vi "Perform Action.vi"(8 "error in":errorcluster, 10 "Input":variant, 11 "AI DAQmx Cont CFG in":refnum<class "AI Current DAQmx Cont CFG.lvclass">) -> (0 "error out":errorcluster, 2 "Output":variant, 3 "AI DAQmx Cont CFG out":refnum<class "AI Current DAQmx Cont CFG.lvclass">)   [LabVIEW 2023, in "AI Current DAQmx Cont CFG.lvclass"]
uses:
  AI Current DAQmx Cont CFG.lvclass
  D:/git/HAL/HAL GOOP4/Configuration/Configuration Semaphore/CFG Semaphore.lvclass
  D:/git/HAL/HAL GOOP4/DAQmx/DAQmx BufferLastReadsDBL/DAQmx BufferLastReadsDBL.lvclass
  D:/git/HAL/HAL GOOP4/DAQmx/DAQmx Base CFG/DAQmx Base CFG.lvclass
  Configuration/Configuration Semaphore/CFG Semaphore.lvclass/CFG Semaphore.ctl
  DAQmx/DAQmx BufferLastReadsDBL/DAQmx BufferLastReadsDBL.lvclass/DAQmx BufferLastReadsDBL.ctl
  DAQmx/DAQmx Base CFG/DAQmx Base CFG.lvclass/DAQmx Base CFG.ctl
  b39270a5-b1fd-40eb-856a-27ea7d92f2a4.vi
  <vilib>/DAQmx/read.llb/DAQmx Read (Analog 2D DBL NChan NSamp).vi
  <vilib>/JDP Science/JSONtext/Find Item.vi
  <vilib>/JDP Science/JSONtext/Next JSON Value.vi
  <vilib>/JDP Science/JSONtext/String Subset.vi
  <vilib>/JDP Science/JSONtext/Parsing/Advance past next JSON Value (inlined COPY).vi
  <vilib>/JDP Science/JSONtext/Parsing/Advance past whitespace.vi
  <vilib>/JDP Science/JSONtext/Parsing/Advance past String.vi
  <vilib>/JDP Science/JSONtext/Parsing/Advance past Number.vi
  <vilib>/JDP Science/JSONtext/Parsing/Advance past Line Ending.vi
  <vilib>/JDP Science/JSONtext/Parsing/Parse Full Path or Item Name.vi
  <vilib>/JDP Science/JSONtext/Parsing/Advance past Array.vi
  <vilib>/JDP Science/JSONtext/Parsing/Advance past Object.vi
  <vilib>/JDP Science/JSONtext/support/Error Cluster From Code.vi
  <vilib>/JDP Science/JSONtext/Offset/Find Item Locations by Path.vi
  <vilib>/JDP Science/JSONtext/JSON text to Variant.vi
  <vilib>/DAQmx/miscellaneous.llb/DAQmx Fill In Error Info.vi
  <vilib>/JDP Science/JSONtext/LVClass Serializer/JSONtext LVClass Serializer.lvclass
  AI Current DAQmx Cont CFG.lvclass/AI Current DAQmx Cont CFG.ctl
  DAQmx/DAQmx Base CFG/DAQmx Base CFG.lvclass
  Configuration/Configuration Semaphore/CFG Semaphore.lvclass
  DAQmx/DAQmx BufferLastReadsDBL/DAQmx BufferLastReadsDBL.lvclass
  DAQmx/BufferLastReadingsDBL/BufferLastReadsDBL.lvclass
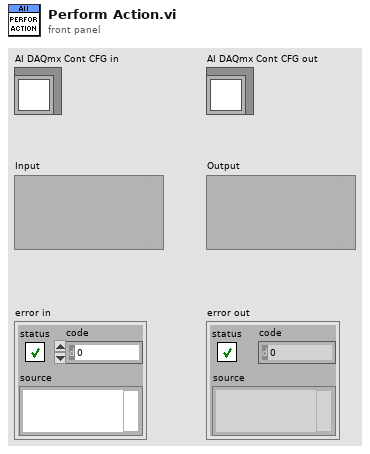
[diagram p1: front panel]
types:
  T1 = typedef "Semaphore RefNum" = refnum<k1>
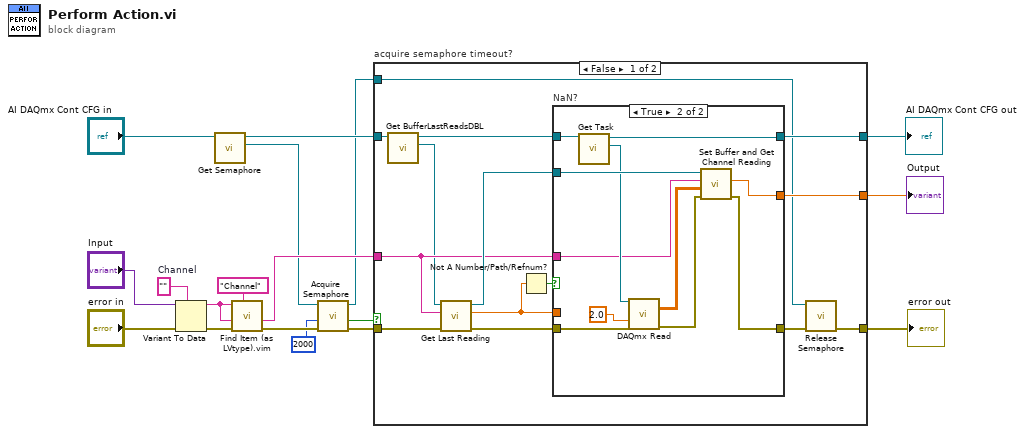
[diagram p0: block diagram]
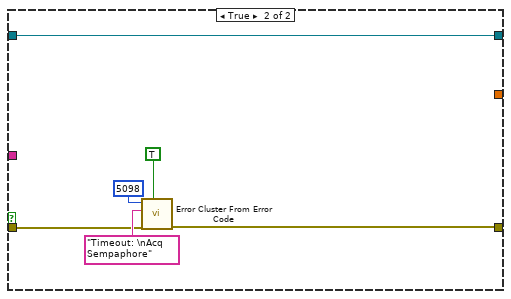
[diagram p3: hidden frame]
diagram:
  w13 = ""  # Channel
  n1 = Variant To Data(error in="error in", type=w13, Variant="Input") -> (data=w10:string, error out=w11:errorcluster)
  n2 = call "Get Semaphore.vi"("CFG Base in"="AI DAQmx Cont CFG in") -> ("Semaphore"=w5:T1, "CFG Base out"=w7:refnum<class "AI Current DAQmx Cont CFG.lvclass">)  [unwired: 9 in]
  n3 = call "Find Item (as LVtype).vim"("$Path or Item Name"="Channel", "error in (no error)"=w11, "Data Type and Default Value"=w10, "JSON"=w10) -> ("error out"=w12:errorcluster, "Data"=w8:string)  [unwired: 4 in, 2 out]
  n4 = call <vilib>:"Acquire Semaphore.vi"("error in (no error)"=w12, "ms timeout (-1)"=2000, "semaphore"=w5) -> ("error out"=w6:errorcluster, "timed out"=w2:bool, "semaphore out"=w1:T1)  [unwired: 2 in]
  n5 = case "acquire semaphore timeout?" shown="False" w2 {
    tunnel: [w20 w48] -> w16
    tunnel: [w30 _] -> w15
    tunnel: w8 -> [w26 _]
    tunnel: w7 -> [w23 w49]
    tunnel: w6 -> [w22 w50]
    tunnel: [w21 w49] -> w3
    tunnel: w1 -> [w19 _]
    frame False {
      n6 = call "Get BufferLastReadsDBL.vi"("DAQmx BufferLastReadsDBL in"=w23) -> ("BufferLastReadsDBL.lvclass"=w24:refnum<class "BufferLastReadsDBL.lvclass">, "DAQmx BufferLastReadsDBL out"=w25:refnum<class "AI Current DAQmx Cont CFG.lvclass">)  [unwired: 9 in]
      n7 = call "Get Last Reading.vi"("error in"=w22, "Channel"=w26, "BufferLastReadingsDBL in"=w24) -> ("error out"=w28:errorcluster, "Reading"=w29:dbl, "BufferLastReadingsDBL out"=w27:refnum<class "BufferLastReadsDBL.lvclass">)  [unwired: 6 in]
      n8 = Not A Number/Path/Refnum?(number/path/refnum=w29) -> (NaN/Path/Refnum?=w31:bool)
      n9 = case "NaN?" shown="True" w31 {
        tunnel: [w33 w43] -> w32
        tunnel: [w34 w40] -> w21
        tunnel: w25 -> [w34 w38]
        tunnel: w27 -> [_ w46]
        tunnel: [w35 w39] -> w30
        tunnel: w29 -> [w35 _]
        tunnel: w28 -> [w33 w42]
        tunnel: w26 -> [_ w41]
        frame False {
        }
        frame True {
          n10 = call "Get Task.vi"("DAQmx Base CFG in"=w38) -> ("Task"=w45:refnum<k21>, "DAQmx Base CFG out"=w40:refnum<class "AI Current DAQmx Cont CFG.lvclass">)  [unwired: 9 in]
          n11 = call-poly <vilib>:"DAQmx Read.vi"("task/channels in"=w45, "timeout"=2.0, "error in"=w42) -> ("data"=w44:dbl[][], "error out"=w36:errorcluster)  [unwired: 10 in, 1 out]
          n12 = call "Set Buffer and Get Channel Reading.vi"("error in"=w36, "Readings"=w44, "Channel Ident"=w41, "BufferLastReadingsDBL in"=w46) -> ("error out"=w43:errorcluster, "Reading"=w39:dbl)  [unwired: 5 in, 1 out]
        }
      }
      n13 = call <vilib>:"Release Semaphore.vi"("error in (no error)"=w32, "semaphore"=w19) -> ("error out"=w20:errorcluster)  [unwired: 4 in, 1 out]
    }
    frame True {
      n14 = call <vilib>:"Error Cluster From Error Code.vi"("show call chain? (False)"=TRUE, "error in (no error)"=w50, "error message (\"\")"="Timeout: \nAcq Sempaphore" ("error message (\"\")"), "error code (0)"=5098) -> ("error out"=w48:errorcluster)  [unwired: 5 in]
    }
  }
  "error out" <- w16
  "AI DAQmx Cont CFG out" <- w3
  "Output" <- w15
